vi "Write rotatorFrame.vi"(8 "error in (no error)":errorcluster, 10 "rotatorFrame":T1, 11 "Rotator in":refnum<class "Rotator.lvclass">) -> (0 "error out":errorcluster, 3 "Rotator out":refnum<class "Rotator.lvclass">)   [LabVIEW 2022 SP3, in "TCSDataDefinitions.lvlib" / "TCSCommand.lvlib" / "TargetConfiguration.lvlib" / "Rotator.lvclass"]
uses:
  Rotator.lvclass
  RotatorCommands/Enumerations/RotatorFrameValues.ctl
  Rotator.lvclass/Rotator.ctl
  TCSCommand.lvlib
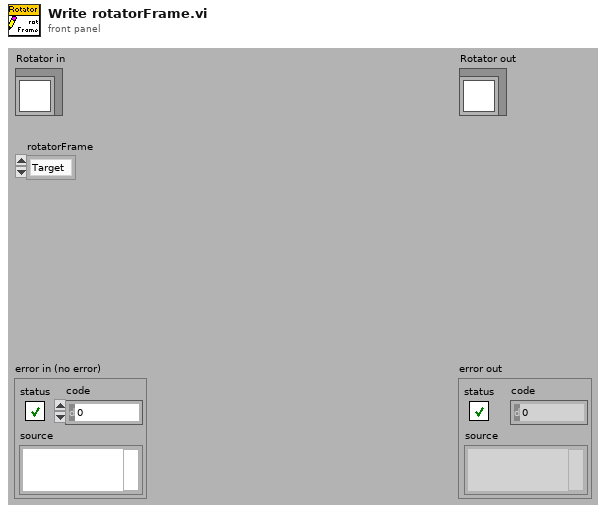
[diagram p1: front panel]
types:
  T1 = typedef "TCSDataDefinitions.lvlib/TCSCommand.lvlib/RotatorFrameValues.ctl" = enum16{"Target", "Fixed"}
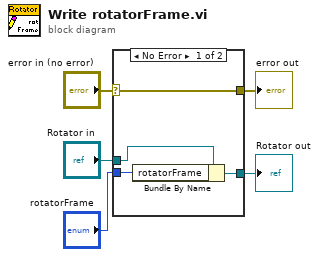
[diagram p0: block diagram]
diagram:
  n1 = case shown="No Error" "error in (no error)" {
    selector: "error in (no error)" -> [w9 w10]
    tunnel: [w9 w10] -> w4
    tunnel: [w7 w11] -> w2
    tunnel: "Rotator in" -> [w8 w11]
    tunnel: "rotatorFrame" -> [w6 _]
    frame No Error {
      n2 = Bundle By Name(cluster=w8, "rotatorFrame"=w6) -> (w7:refnum<class "Rotator.lvclass">)
    }
    frame Error {
    }
  }
  "error out" <- w4
  "Rotator out" <- w2
